vi "_015.vi"() -> ()   [LabVIEW 2024]
panel:
  in  "Cluster":cluster{"Numeric":dbl}
  out "Boolean":bool
  out "Numeric 4":i32
  out "Numeric 3":i32
  out "input":dbl
  out "output":dbl
  out "S":dbl
  out "Iteration Count":dbl
  in  "Numeric 2":dbl
  in  "stop":bool
  out "Numeric":dbl
  # "Shift Register ( operations ) :"
  # "previous val"
  # "2 times previous val"
  # "3 times previous val"
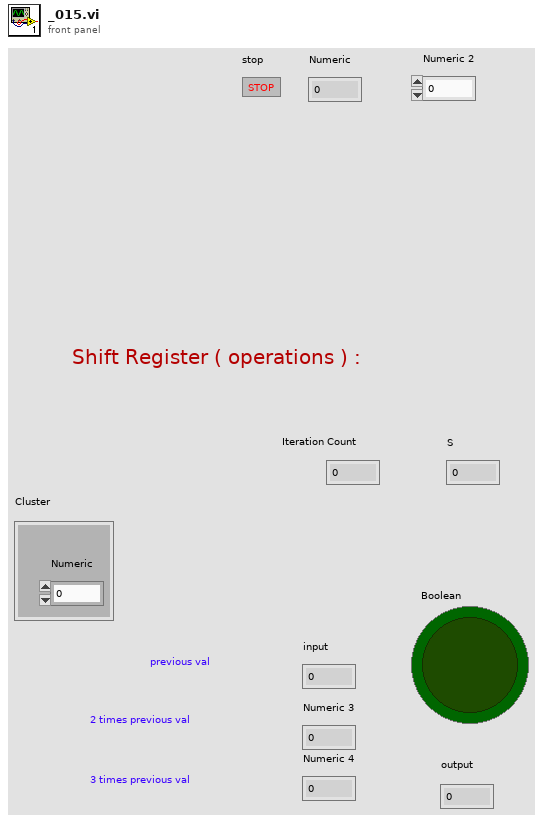
[diagram p1: front panel]
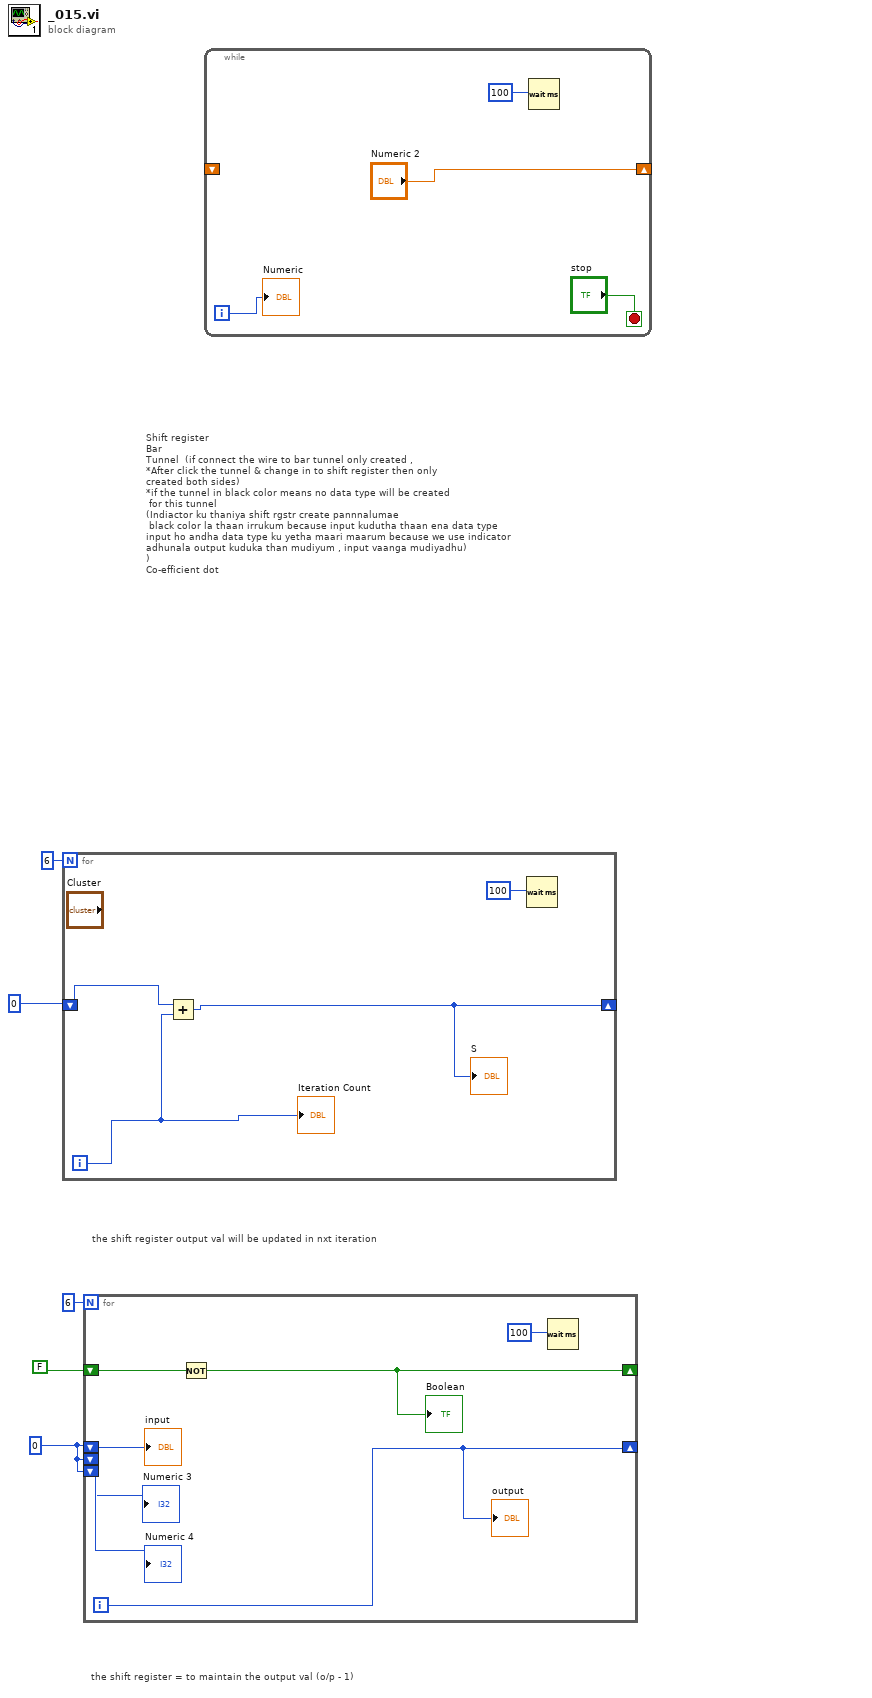
[diagram p0: block diagram]
diagram:
  w2 = 0
  # "the shift register = to maintain the output val (o/p - 1)"
  # "the shift register output val will be updated in nxt iteration"
  # "Shift register\nBar \nTunnel  (if connect the wire to bar tunnel only created , \n*After click the tunnel & change in to shift register then only \ncreated both sides)\n*if the tunnel in black color means no data type will be created\n for this tunnel\n(Indiactor ku thaniya shift rgstr create pannnalumae\n black color la thaan irrukum because input kudutha thaan ena data type\ninput ho andha data type ku yetha maari maarum because we use indicator\nadhunala output kuduka than mudiyum , input vaanga mudiyadhu) \n)\nCo-efficient dot"
  n1 = for {
    N: 6 -> [_]
    shift-right: [w6] -> _
    shift-left: 0 -> [w7]
    i -> [w8]
    n2 = Add(x=w7, y=w8) -> (x+y=w6:i32)
    "S" <- w6
    n3 = Wait (ms)(milliseconds to wait=100) -> ()  [unwired: 1 out]
    "Iteration Count" <- w8
  }
  n4 = for {
    N: 6 -> [_]
    shift-right: [w14] -> _
    shift-left: w2 -> [w15]
    shift-left: w2 -> [w12]
    shift-left: w2 -> [w13]
    shift-right: [w10] -> _
    shift-left: FALSE -> [w11]
    i -> [w14]
    n5 = Not(x=w11) -> (.not. x?=w10:bool)
    "Boolean" <- w10
    n6 = Wait (ms)(milliseconds to wait=100) -> ()  [unwired: 1 out]
    "output" <- w14
    "input" <- w15
    "Numeric 3" <- w12
    "Numeric 4" <- w13
  }
  n7 = while {
    shift-right: ["Numeric 2"] -> _
    shift-left: _ -> [_]
    i -> [w19]
    stop <- "stop" stop-if-true
    n8 = Wait (ms)(milliseconds to wait=100) -> ()  [unwired: 1 out]
    "Numeric" <- w19
  }
